vi "TTLPreparation_171213.vi"(11 "TTLArray":T1(array[cluster])) -> ()   [LabVIEW 2016]
uses:
  Globaltracker.vi
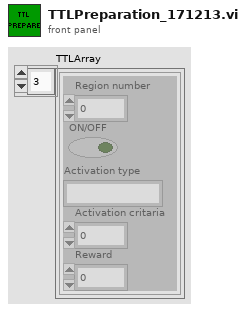
[diagram p1: front panel]
types:
  T1 = cluster{"Region number":i32, "ON/OFF":bool, "Activation type":string, "Activation critaria":i32, "Reward":i32}[]
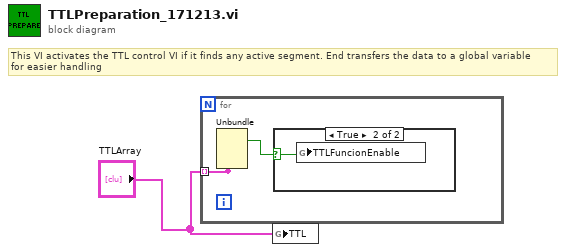
[diagram p0: block diagram]
diagram:
  # "This VI activates the TTL control VI if it finds any active segment. End transfers the data to a global variable \nfor easier handling"
  n1 = for {
    tunnel: [w2] -> _ mode=indexing
    tunnel: "TTLArray" -> [w2] mode=indexing
    n2 = Unbundle(w2) -> ("ON/OFF"=w3:bool)  [unwired: 4 out]
    n3 = case shown="True" w3 {
      selector: w3 -> [_ w4]
      frame False {
      }
      frame True {
        n4 = global write "Globaltracker.vi" "TTLFuncionEnable"(w4) -> ()
      }
    }
  }
  n5 = global write "Globaltracker.vi" "TTL"("TTLArray") -> ()
